vi "flow-builder.water-temp-dosing.vi"(7 "Proc Name":string="EC", 8 "error in":errorcluster, 9 "Unit Index":i32, 11 "Nutrition Cluster":T3 {"ORP Dosing"."MIX Limit" format="%d [s]"; "ORP Dosing"."MIX Dose" format="%d [s]"; "PH Dosing"."ACID Limit" format="%d [s]"; "PH Dosing"."BASE Limit" format="%d [s]"; "PH Dosing"."ACID Dose" format="%d [s]"; "PH Dosing"."BASE Dose" format="%d [s]"; "EC Dosing"."BETA2 Limit" format="%d [s]"; "EC Dosing"."ALFA2 Limit" format="%d [s]"; "EC Dosing"."ALFA2 Dose" format="%d [s]"; "EC Dosing"."BETA2 Dose" format="%d [s]"; "EC Dosing"."BETA1 Limit" format="%d [s]"; "EC Dosing"."ALFA1 Limit" format="%d [s]"; "EC Dosing"."ALFA1 Dose" format="%d [s]"; "EC Dosing"."BETA1 Dose" format="%d [s]"; "Main"."DailyActivityHours"."Begin Time" format="ON:    %<%H:%M>T"; "Main"."DailyActivityHours"."End Time" format="OFF:    %<%H:%M>T"; "Main"."WashTimes"."Out" format="Wash out: %d [sec]"; "Main"."WashTimes"."In" format="Wash in: %d [sec]"; "Water Dosing"."Water Limit" format="%d [s]"; "Water Dosing"."Water Dose" format="%d [s]"}) -> (0 "error out":errorcluster, 1 "WillDose?":bool, 2 "status":string, 3 "Flow out":T1[](array[typedef]))   [LabVIEW 2024]
uses:
  controls/UiNutritionPanel.ctl
  controls/UiScheduleTimestamp.ctl
  controls/UiStepBuilder.ctl
  controls/type.step-builder.ctl
  io.interface.serial.vi
  <vilib>/Utility/error.llb/Trim Whitespace One-Sided.vi
  <vilib>/Utility/error.llb/Clear Errors.vi
  Polymorphics/variantCtrlIo.vi
  globals/globals-engine.vi
  util.environment.vi
  util-address-parser.vi
  util-address-builder.vi
  util.DO.ToString.vi
  Polymorphics/io.command-builder.vi
  Polymorphics/io.command-builder.DO.vi
  Polymorphics/io.command-builder.AI.vi
  Polymorphics/io.command-builder.DI.vi
  io.frame.vi
  io.visa.vi
  io.responseValidator.vi
  Polymorphics/io.command-parser.DI.vi
  Polymorphics/io.command-parser.AI.vi
panel:
  out "Dosing Tabel":cluster{"Dose Time":dbl, "Input":string}[](array[cluster])
  in  "simulator":dbl=3.0
  out "Low Range":bool
  out "Low Alarm":bool
  out "High Alarm":bool
  # "Water"
  # "EC"
  # "PH"
  # "ORP"
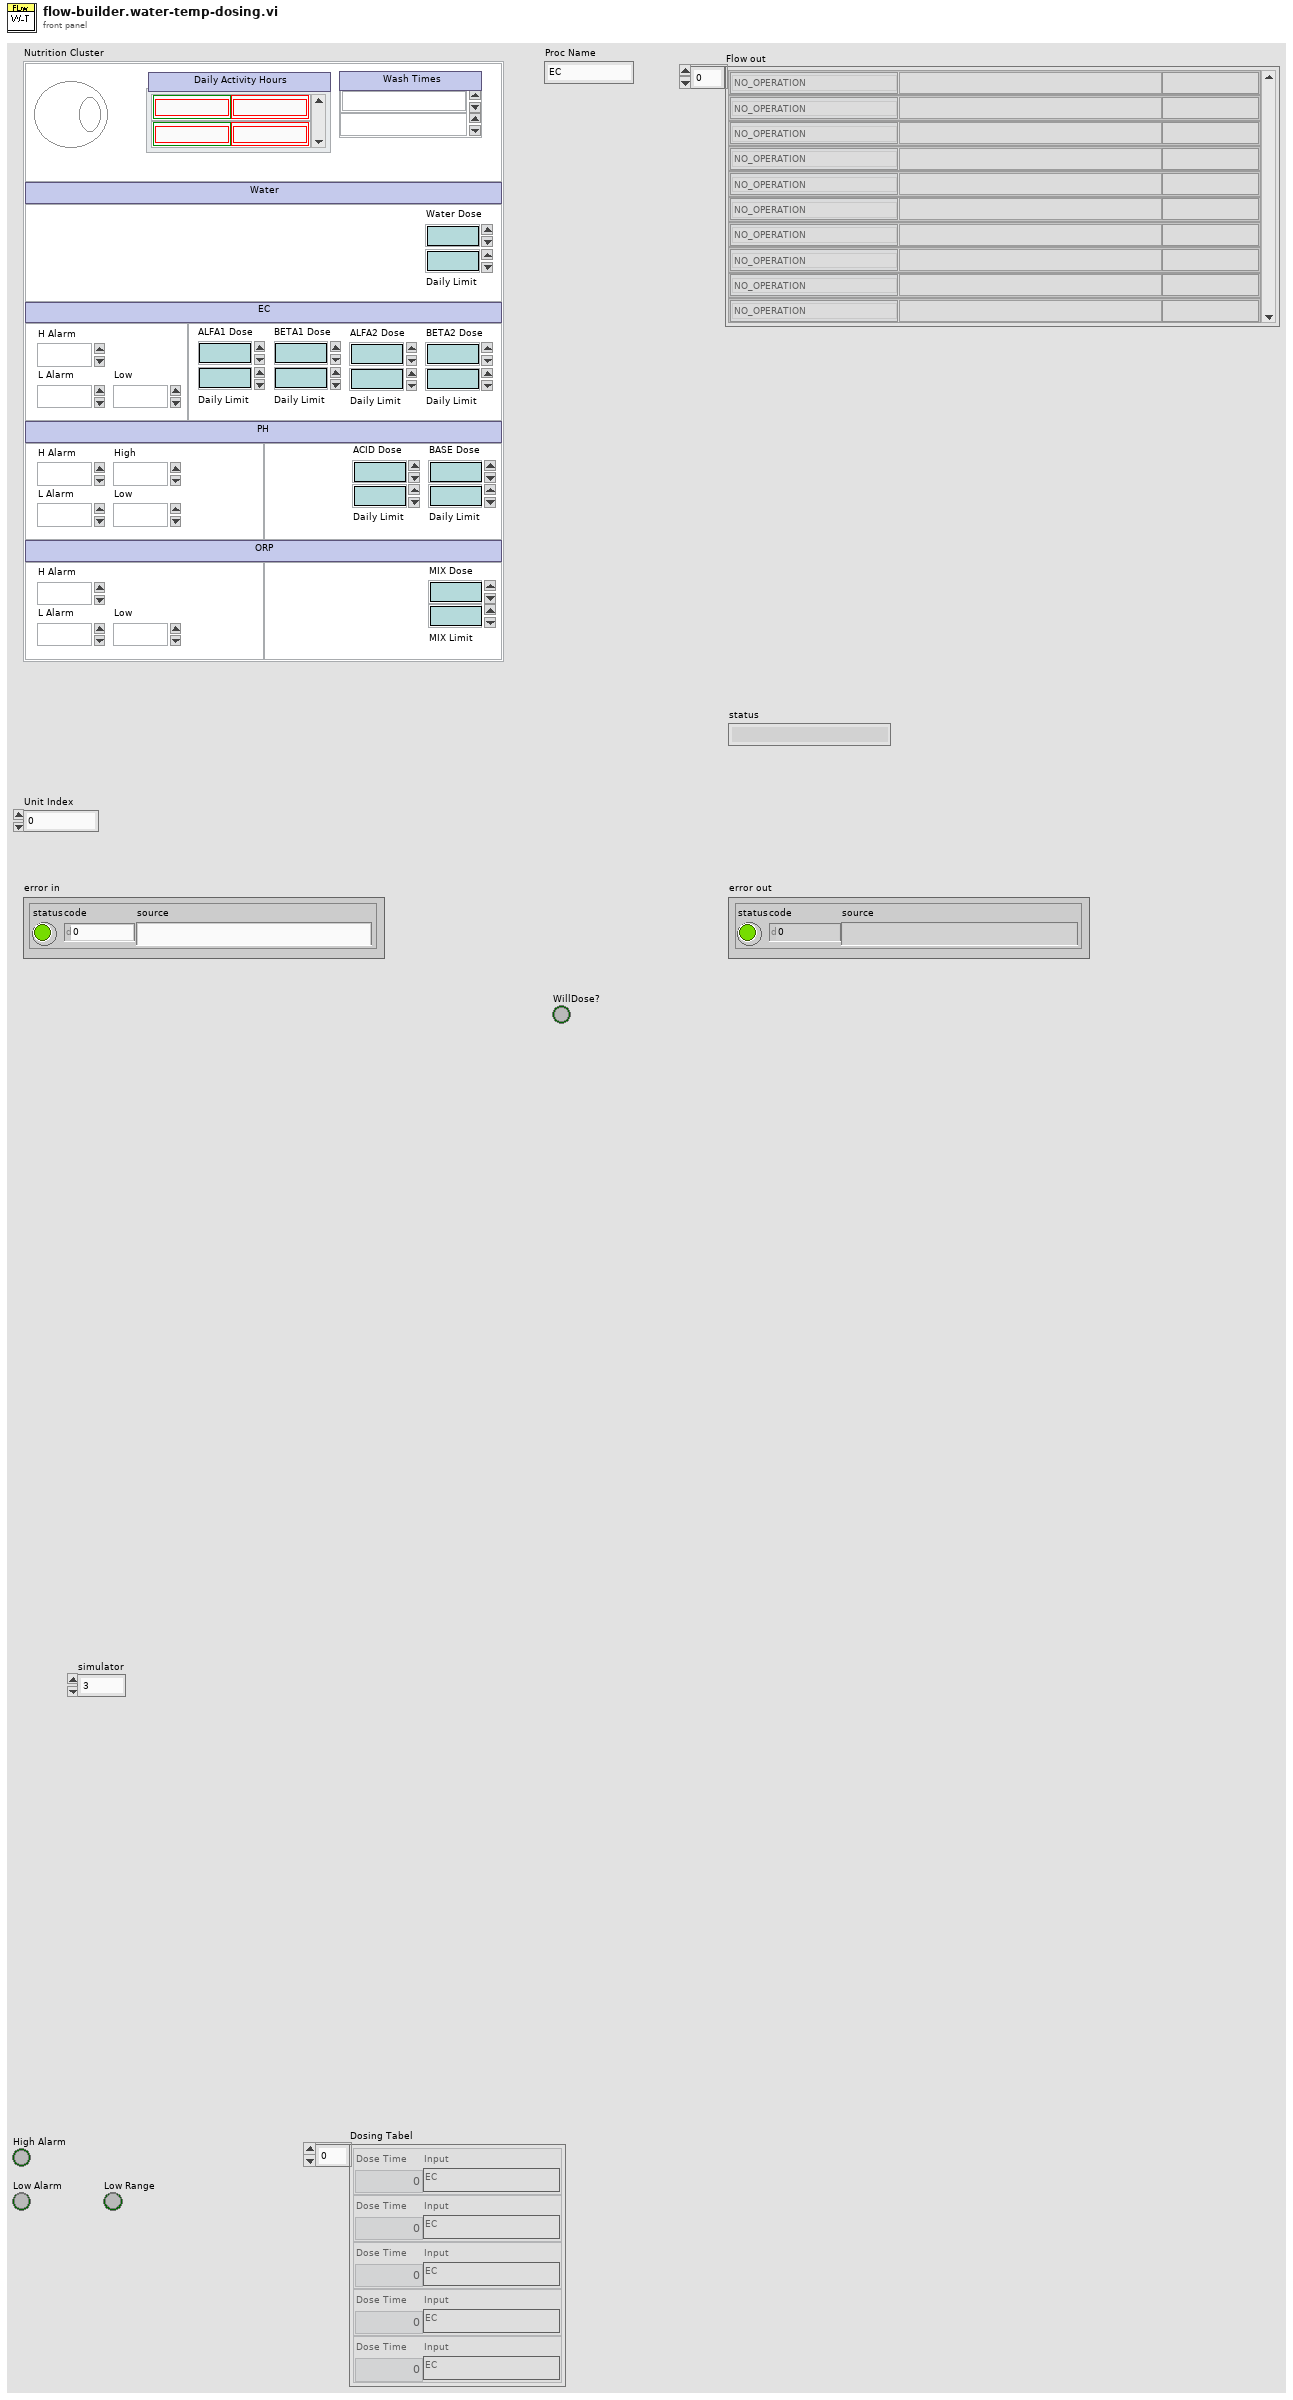
[diagram p1: front panel]
types:
  T1 = typedef "UiStepBuilder.ctl" = cluster{"Step Function":T2, "ParamString":string, "Step Label":string}
  T2 = typedef "type.step-builder.ctl" = enum16{"NO_OPERATION", "DELAY-JUMP", "DELAY", "JUMP", "COMPLETE", "SCHEDULER", "IRR-CHECK", "UNIT-CHECK", "UNIT-SAMPLE", "UNIT-DOSE", "LOG-REPORT", "LOG-MESSAGE", "IO-READ", "IO-READ-MANY", "IO-WRITE", "IO-COMPARE-OUT", "IO-COMPARE-IN", "PROC-START", "PROC-STOP", "PROC-LOAD", "PROC-IS-COMPLETED", "RECORD-MOVE", "GET-RH", "GET-UV", "GET-WD", "GET-WS", "OCS-CHECK", "OCS-RECORD"}
  T3 = typedef "UiNutritionPanel.ctl" = cluster{"Main":cluster{"Enable":bool, "WashTimes":cluster{"In":dbl, "Out":dbl}, "DailyActivityHours":cluster{"Begin Time":T4, "End Time":T4}[]}, "Water Dosing":cluster{"Water Dose":dbl, "Water Limit":dbl}, "EC Ranges":cluster{"H Alarm":dbl, "L Alarm":dbl, "Low":dbl}, "EC Dosing":cluster{"ALFA1 Dose":dbl, "ALFA1 Limit":dbl, "BETA1 Dose":dbl, "BETA1 Limit":dbl, "ALFA2 Dose":dbl, "ALFA2 Limit":dbl, "BETA2 Dose":dbl, "BETA2 Limit":dbl}, "PH Ranges":cluster{"H Alarm":dbl, "L Alarm":dbl, "High":dbl, "Low":dbl}, "PH Dosing":cluster{"ACID Dose":dbl, "ACID Limit":dbl, "BASE Dose":dbl, "BASE Limit":dbl}, "ORP Ranges":cluster{"H Alarm":dbl, "L Alarm":dbl, "Low":dbl}, "ORP Dosing":cluster{"MIX Dose":dbl, "MIX Limit":dbl}}
  T4 = typedef "UiScheduleTimestamp.ctl" = timestamp
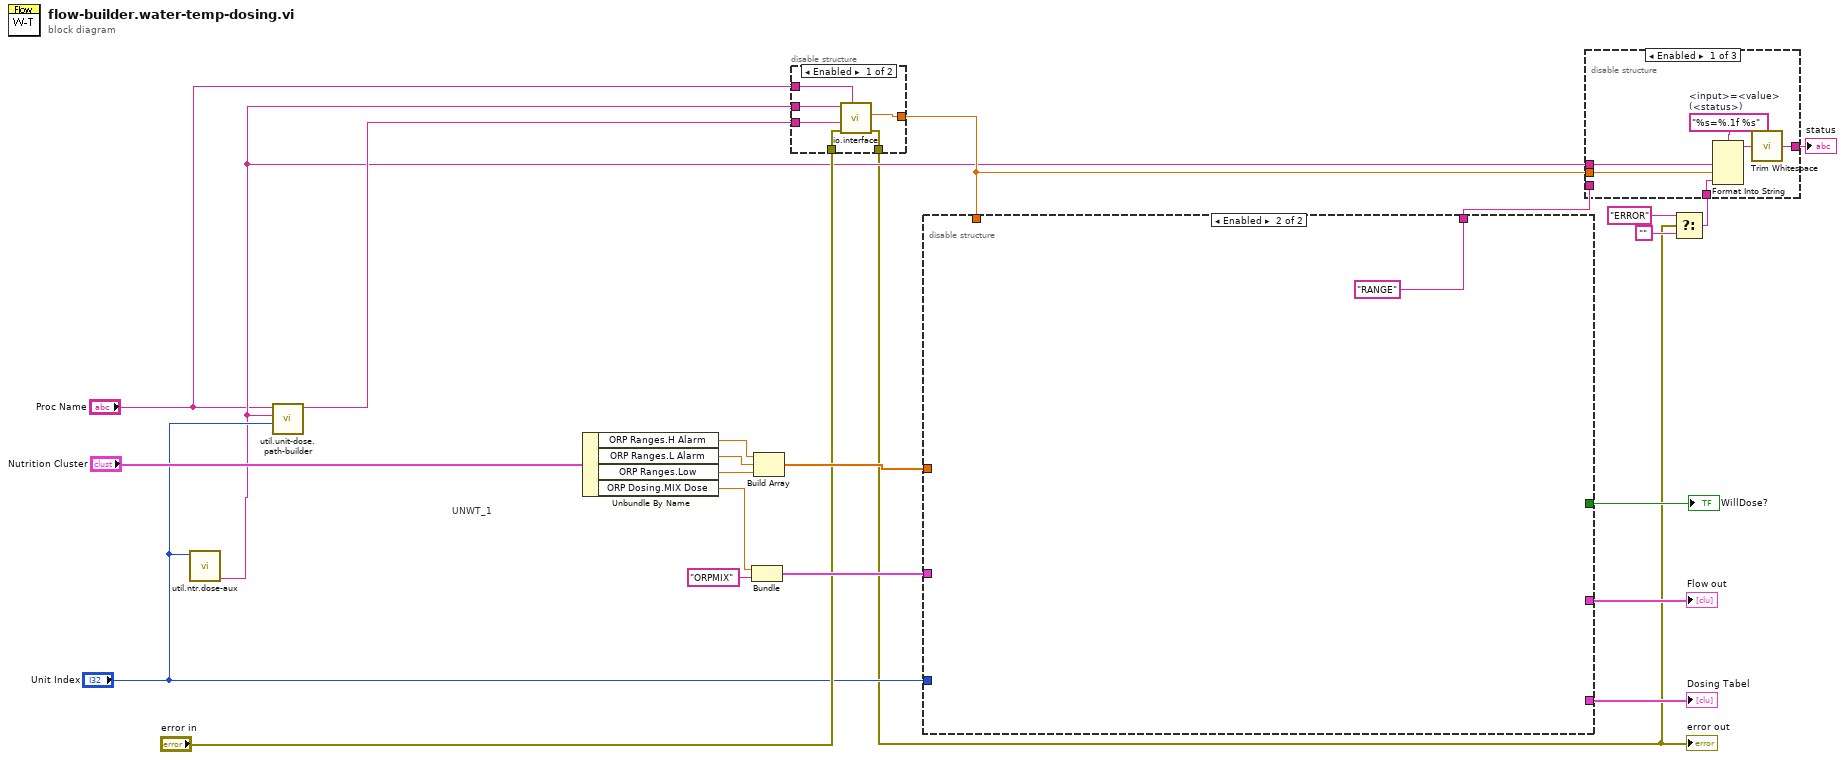
[diagram p0: block diagram]
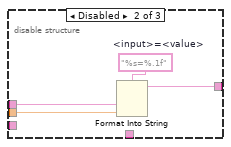
[diagram p2: hidden frame]
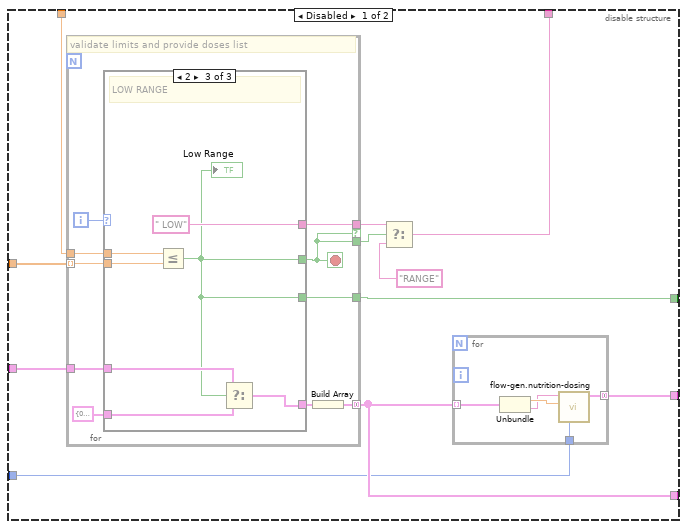
[diagram p4: hidden frame]
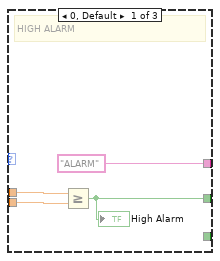
[diagram p5: hidden frame]
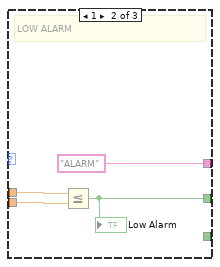
[diagram p6: hidden frame]
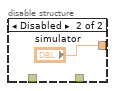
[diagram p7: hidden frame]
diagram:
  # "UNWT_1"
  n1 = call "util.ntr.dose-aux.vi"("Unit Index"="Unit Index") -> ("Unit Water Temperature (UN_WT)"=w7:string)  [unwired: 6 in, 4 out]
  n2 = call "util.unit-dose.path-builder.vi"("Unit Index"="Unit Index", "Input"=w7, "Proc Name"="Proc Name") -> ("\\NUTRITION\\ORP\\ORP_U1_2024-08-16.*"=w11:string)  [unwired: 8 in]
  n3 = Unbundle By Name("Nutrition Cluster") -> ("ORP Ranges.H Alarm"=w23:dbl, "ORP Ranges.L Alarm"=w21:dbl, "ORP Ranges.Low"=w20:dbl, "ORP Dosing.MIX Dose"=w16:dbl)
  n4 = Bundle("MIX Dose"=w16, "I/O"="ORPMIX") -> (w15:cluster{"MIX Dose":dbl, "I/O":string})  [unwired: 1 in]
  n5 = Build Array(w23, w21, w20) -> (w22:dbl[])
  n6 = disable-structure shown="Enabled" {
    disable-tunnel: w7 -> [w29 _]
    disable-tunnel: [w28 "simulator"] -> w10
    disable-tunnel: [w27 _] -> w3
    disable-tunnel: "error in" -> [w26 _]
    disable-tunnel: w11 -> [w25 _]
    disable-tunnel: "Proc Name" -> [w24 _]
    frame Enabled {
      n7 = call "io.interface.vi"("Caller"=w24, "error in"=w26, "record filename.* (disabled if empty)"=w25, "IO Name in"=w29) -> ("error out"=w27:errorcluster, "Value out"=w28:dbl)  [unwired: 2 in, 4 out]
    }
    frame Disabled {
    }
  }
  "error out" <- w3
  n8 = disable-structure shown="Enabled" {
    disable-tunnel: w22 -> [w41 _]
    disable-tunnel: [w40 _] -> w18
    disable-tunnel: [w39 _] -> w17
    disable-tunnel: w15 -> [w38 _]
    disable-tunnel: "Unit Index" -> [w37 _]
    disable-tunnel: w10 -> [w33 _]
    disable-tunnel: [w32 "RANGE"] -> w6
    disable-tunnel: [w31 _] -> w9
    frame Disabled {
      n9 = for {
        tunnel: w41 -> [w55] mode=indexing
        tunnel: [w54] -> w35 if=w52
        tunnel: w33 -> [w53]
        tunnel: [w52] -> w36
        tunnel: [w50] -> w40 mode=concatenating
        tunnel: w38 -> [w49]
        tunnel: [w47] -> w31
        i -> [w56]
        stop <- w52 stop-if-true
        # "validate limits and provide doses list"
        n10 = case shown="2" w56 {
          tunnel: w55 -> [w59 w63 w70]
          tunnel: [w57 w61 w65] -> w52
          tunnel: ["ALARM" "ALARM" " LOW"] -> w54
          tunnel: w53 -> [w58 w62 w69]
          tunnel: [_ _ w68] -> w51
          tunnel: w49 -> [_ _ w66]
          tunnel: cluster{"BETA-2":dbl, "I/O":string} {"BETA-2"=0.0, "I/O"=""} ("f") -> [_ _ w67]
          tunnel: [_ _ w65] -> w47
          frame 0, Default {
            # "HIGH ALARM"
            n11 = Greater Or Equal?(x=w58, y=w59) -> (x >= y?=w57:bool)
            "High Alarm" <- w57
          }
          frame 1 {
            # "LOW ALARM"
            n12 = Less Or Equal?(x=w62, y=w63) -> (x <= y?=w61:bool)
            "Low Alarm" <- w61
          }
          frame 2 {
            # "LOW RANGE"
            n13 = Less Or Equal?(x=w69, y=w70) -> (x <= y?=w65:bool)
            "Low Range" <- w65
            n14 = Select(t=w66, s=w65, f=w67) -> (s? t:f=w68:cluster{"BETA-2":dbl, "I/O":string})
          }
        }
        n15 = Build Array(w51) -> (w50:cluster{"BETA-2":dbl, "I/O":string}[])
      }
      n16 = Select(t=w35, s=w36, f="RANGE") -> (s? t:f=w32:string)
      n17 = for {
        tunnel: [w46] -> w39 mode=concatenating
        tunnel: w40 -> [w45] mode=indexing
        tunnel: w37 -> [w42]
        n18 = Unbundle(w45) -> ("BETA-2"=w44:dbl, "I/O"=w43:string)
        n19 = call "flow-gen.nutrition-dosing.vi"("Unit Index"=w42, "Dosing Time"=w44, "IO Name"=w43) -> ("Flow"=w46:T1[])  [unwired: 7 in, 1 out]
      }
    }
    frame Enabled {
    }
  }
  "Flow out" <- w17
  "Dosing Tabel" <- w18
  "WillDose?" <- w9
  n20 = Select(t="ERROR", s=w3, f="") -> (s? t:f=w2:string)
  n21 = disable-structure shown="Enabled" {
    disable-tunnel: [w73 w82 _] -> w13
    disable-tunnel: w10 -> [w76 w80 _]
    disable-tunnel: w7 -> [w75 w79 _]
    disable-tunnel: w6 -> [_ _ _]
    disable-tunnel: w2 -> [w74 _ _]
    frame Enabled {
      w77 = "%s=%.1f %s"  # <input>=<value> (<status>)
      n22 = Format Into String(format string=w77, w75, w76, w74) -> (resulting string=w78:string)  [unwired: 2 in, 1 out]
      n23 = call <vilib>:"Trim Whitespace.vi"("string"=w78) -> ("trimmed string"=w73:string)  [unwired: 1 in]
    }
    frame Disabled {
      w81 = "%s=%.1f"  # <input>=<value>
      n24 = Format Into String(format string=w81, w79, w80) -> (resulting string=w82:string)  [unwired: 2 in, 1 out]
    }
    frame Disabled {
    }
  }
  "status" <- w13
